vi "Init Module.vi"(8 "error in (no error)":errorcluster, 11 "Singleton Module Admin in":refnum<class "Delacor_lib_QMH_Module Admin.lvclass">) -> (0 "error out":errorcluster, 2 "FlexiFlowInterface Request Events":T1, 3 "Singleton Module Admin out":refnum<class "Delacor_lib_QMH_Module Admin.lvclass">)   [LabVIEW 2024, in "FlexiFlowInterface.lvlib"]
doc: "Initialize the module by creating Broadcast Events, Request Events, and synchronization rendezvous.\n_____\nBased on Delacor QMH Project Template 3.1.0.34."
uses:
  FlexiFlowInterface.lvlib
  <vilib>/Delacor/Delacor QMH/Libraries/Module Admin_class/Delacor_lib_QMH_Module Admin.lvclass
  Request Events--cluster.ctl
  Stop Argument--cluster.ctl
  Show Panel Argument--cluster.ctl
  Hide Panel Argument--cluster.ctl
  Get Module Execution Status Argument--cluster.ctl
  Show Diagram Argument--cluster.ctl
  Change Panel Argument--cluster.ctl
  <vilib>/MGI/Panel Manager/Panel/Panel/Panel.lvclass
  Start Modbus Polling Helper Loop Argument--cluster.ctl
  Sleep Modbus Polling Helper Loop Argument--cluster.ctl
  Wake Connection Helper Loop Argument--cluster.ctl
  Sleep Connection Helper Loop Argument--cluster.ctl
  Initialise Modbus Connections Argument--cluster.ctl
  Read Fmeasure Argument--cluster.ctl
  FlexiFlowDevice--enum.ctl
  Set Modbus Configuration Argument--cluster.ctl
  Modbus TCP Connection Settings--cluster.ctl
  Wink Devices Argument--cluster.ctl
  Read All FlexiFlow Device States Argument--cluster.ctl
  Wink Device Argument--cluster.ctl
  Set Control Function Argument--cluster.ctl
  Modbus Flexi-Flow API/Control Function Values--enum.ctl
  Set Flow Setpoint Argument--cluster.ctl
  Set Backpressure Setpoint Argument--cluster.ctl
  Set Forward Pressure SP Argument--cluster.ctl
  Set Capacity Unit Argument--cluster.ctl
  Capacity unit--text ring.ctl
  Set Flow Capacity Unit Argument--cluster.ctl
  Modbus Flexi-Flow API/Capacity Units (Standard Volume Flow).ctl
  Set Setpoint Slope Argument--cluster.ctl
  Set Counter Settings Argument--cluster.ctl
  Counter Settings--cluster.ctl
  Modbus Flexi-Flow API/Counter Setpoint Mode--enum.ctl
  Modbus Flexi-Flow API/Counter Modes--enum.ctl
  Reset All Device Counters Argument--cluster.ctl
  Read Device User Tag Argument--cluster.ctl
  Set Device User Tag Argument--cluster.ctl
  Read Counter Unit Argument--cluster.ctl
  Set Control Mode Argument--cluster.ctl
  Modbus Flexi-Flow API/Control Mode--enum.ctl
  Get Device Configuration Argument--cluster.ctl
  Modbus Flexi-Flow API/Bronkhorst Flexi-Flow ModbusTCP API.lvlib
  Anode/Anode.lvlib
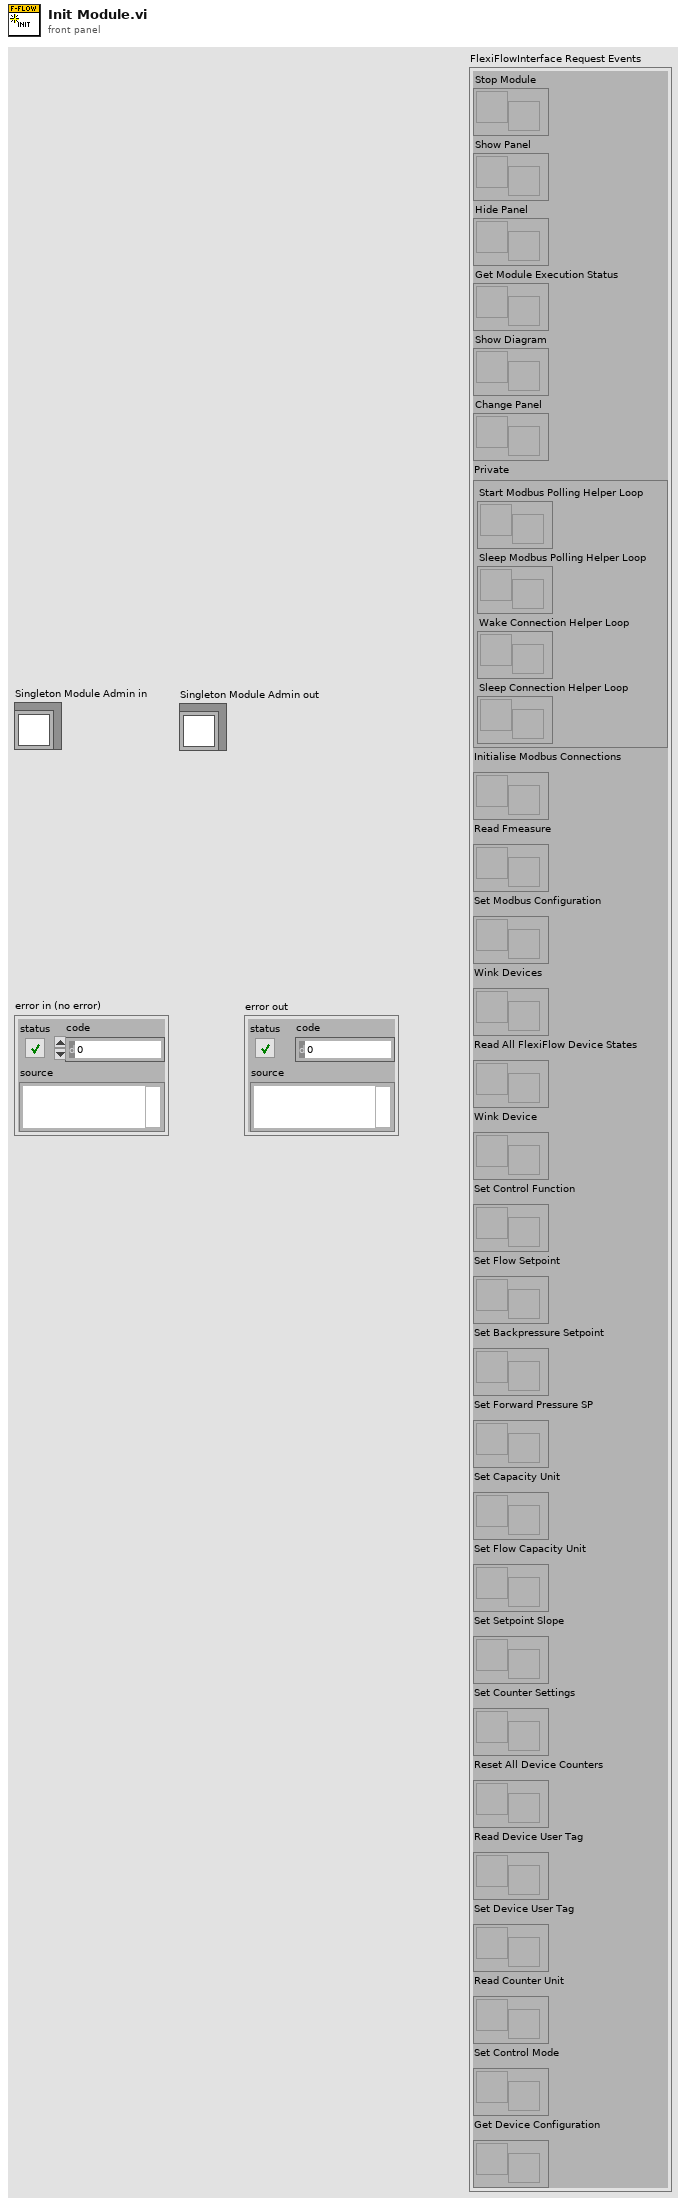
[diagram p1: front panel]
types:
  T1 = typedef "FlexiFlowInterface.lvlib/Request Events--cluster.ctl" = cluster{"Stop Module":refnum<user-event>, "Show Panel":refnum<user-event>, "Hide Panel":refnum<user-event>, "Get Module Execution Status":refnum<user-event>, "Show Diagram":refnum<user-event>, "Change Panel":refnum<user-event>, "Private":cluster{"Start Modbus Polling Helper Loop":refnum<user-event>, "Sleep Modbus Polling Helper Loop":refnum<user-event>, "Wake Connection Helper Loop":refnum<user-event>, "Sleep Connection Helper Loop":refnum<user-event>}, "Initialise Modbus Connections":refnum<user-event>, "Read Fmeasure":refnum<user-event>, "Set Modbus Configuration":refnum<user-event>, "Wink Devices":refnum<user-event>, "Read All FlexiFlow Device States":refnum<user-event>, "Wink Device":refnum<user-event>, "Set Control Function":refnum<user-event>, "Set Flow Setpoint":refnum<user-event>, "Set Backpressure Setpoint":refnum<user-event>, "Set Forward Pressure SP":refnum<user-event>, "Set Capacity Unit":refnum<user-event>, "Set Flow Capacity Unit":refnum<user-event>, "Set Setpoint Slope":refnum<user-event>, "Set Counter Settings":refnum<user-event>, "Reset All Device Counters":refnum<user-event>, "Read Device User Tag":refnum<user-event>, "Set Device User Tag":refnum<user-event>, "Read Counter Unit":refnum<user-event>, "Set Control Mode":refnum<user-event>, "Get Device Configuration":refnum<user-event>}
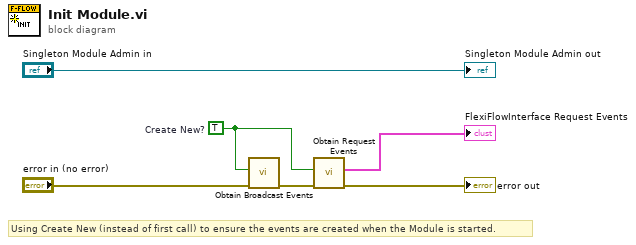
[diagram p0: block diagram]
diagram:
  w3 = TRUE  # Create New?
  # "Using Create New (instead of first call) to ensure the events are created when the Module is started."
  n1 = call "Obtain Broadcast Events.vi"("error in (no error)"="error in (no error)", "Create New?"=w3) -> ("error out"=w6:errorcluster)  [unwired: 8 in, 1 out]
  n2 = call "Obtain Request Events.vi"("error in (no error)"=w6, "Create New?"=w3) -> ("error out"=→"error out":errorcluster, "FlexiFlowInterface Request Events"=→"FlexiFlowInterface Request Events":T1)  [unwired: 8 in]
  "Singleton Module Admin out" <- "Singleton Module Admin in"
